vi "task_2.vi"() -> ()   [LabVIEW 2018]
panel:
  in  "stop":bool
  in  "Slide":dbl(slide) scale=0.0..10.0
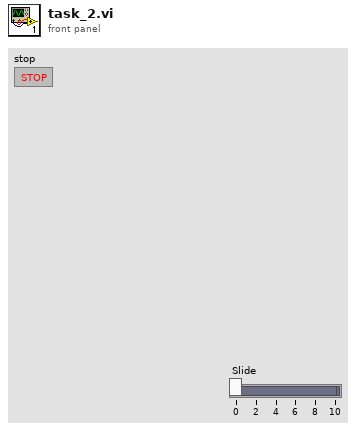
[diagram p1: front panel]
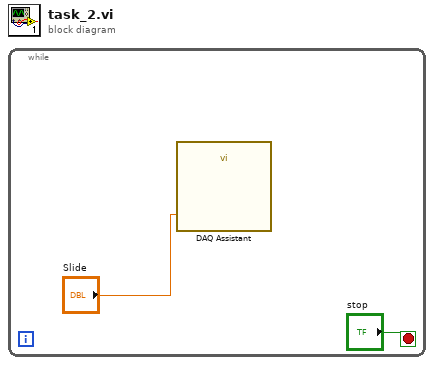
[diagram p0: block diagram]
diagram:
  n1 = while {
    stop <- "stop" stop-if-true
    n2 = call "DAQ Assistant"("data"="Slide") -> ()  [unwired: 17 in, 2 out]
  }
